vi "Priority.vi"(8 "error in (no error)":errorcluster, 11 "QueryAuthController in":refnum<class "QueryAuthController.lvclass">) -> (0 "error out":errorcluster, 2 "Priority":u16, 3 "QueryAuthController out":refnum<class "QueryAuthController.lvclass">)   [LabVIEW 2020]
uses:
  QueryAuthController.lvclass
  QueryAuthController.lvclass/QueryAuthController.ctl
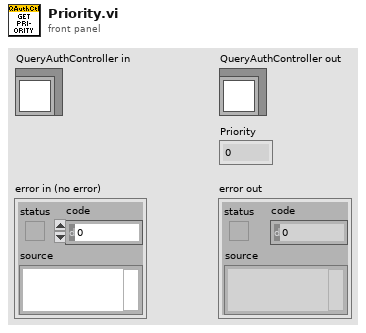
[diagram p1: front panel]
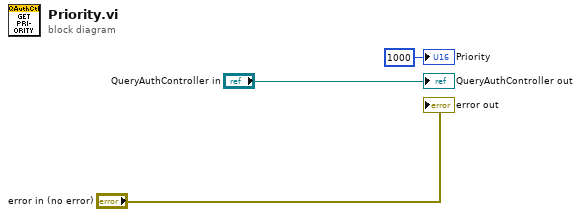
[diagram p0: block diagram]
diagram:
  "error out" <- "error in (no error)"
  "QueryAuthController out" <- "QueryAuthController in"
  "Priority" <- u16 1000 ("Priority")
